vi "XiXi-1(Multify And Boolean[]).vi"(10 "X[-1]":bool[](array[boolean]), 11 "Xi":bool[][](array[boolean])) -> (3 "Yi":bool[][](array[boolean]))   [LabVIEW 2012]
doc: "Calculate sums of consecutive array elements. 0th element of output is equal to x(0)+ x(-1), where x(-1) is an optional scalar input that defaults to zero."
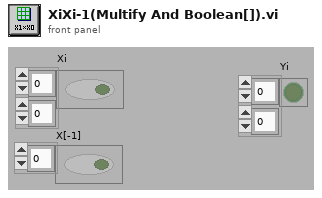
[diagram p1: front panel]
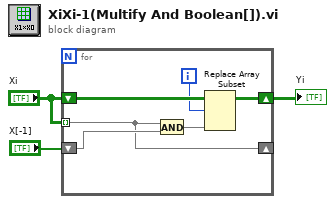
[diagram p0: block diagram]
diagram:
  n1 = for {
    shift-right: [w8] -> w1
    shift-left: "Xi" -> [w9]
    shift-right: [w4] -> _
    shift-left: "X[-1]" -> [w6]
    tunnel: "Xi" -> [w4] mode=indexing
    i -> [w7]
    n2 = And(x=w4, y=w6) -> (x .and. y?=w5:bool[])
    n3 = Replace Array Subset(array=w9, new element=w5, index (row)=w7) -> (w8:bool[][])  [unwired: 1 in]
  }
  "Yi" <- w1
